vi "Finish.vi"(8 "error in (no error)":errorcluster, 11 "Compressor in":refnum<class "Compressor.lvclass">) -> (0 "error out":errorcluster, 3 "Compressor out":refnum<class "Compressor.lvclass">)   [LabVIEW 2013, in "Compressor.lvclass"]
uses:
  Compressor.lvclass
  System/System.lvclass
  Compressor.lvclass/Compressor.ctl
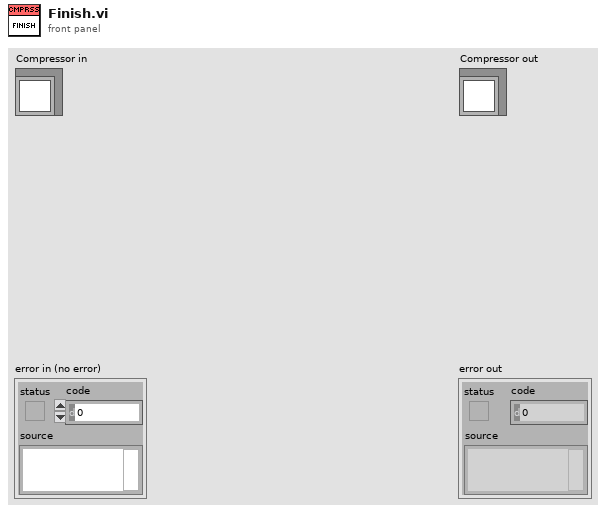
[diagram p1: front panel]
types:
  T1 = typedef "WPI_CompressorDevRef.ctl" = cluster{"DevStatus":errorcluster, "DigitalInputDevRef":T2, "RelayDevRef":T5}
  T2 = typedef "WPI_DigitalInputDevRef.ctl" = cluster{"DevStatus":errorcluster, "DIO Channel":T3, "Digital Module":T4}
  T3 = typedef "FPGA_DIOChannel.ctl" = enum8{"DIO 1", "DIO 2", "DIO 3", "DIO 4", "DIO 5", "DIO 6", "DIO 7", "DIO 8", "DIO 9", "DIO 10", "DIO 11", "DIO 12", "DIO 13", "DIO 14", "Invalid"}
  T4 = typedef "FPGA_TypedefDigitalModule.ctl" = enum16{"Digital Module 1", "Digital Module 2"}
  T5 = typedef "WPI_RelayDevRef.ctl" = cluster{"DevStatus":errorcluster, "Relay Channel":T6, "Digital Module":T4, "Relay Direction":T7}
  T6 = typedef "FPGA_DIORelayChannel.ctl" = enum8{"Relay 1", "Relay 2", "Relay 3", "Relay 4", "Relay 5", "Relay 6", "Relay 7", "Relay 8", "Invalid"}
  T7 = typedef "WPI_RelayDirection.ctl" = enum16{"Both directions", "Forward only", "Reverse only"}
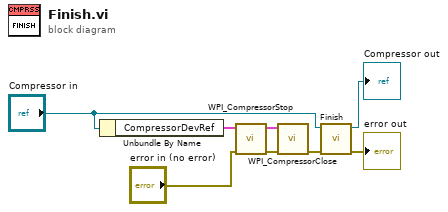
[diagram p0: block diagram]
diagram:
  n1 = Unbundle By Name("Compressor in") -> ("CompressorDevRef"=w3:T1)
  n2 = call <vilib>:"WPI_CompressorStop.vi"("error in (no error)"="error in (no error)", "CompressorDevRef"=w3) -> ("error out"=w6:errorcluster, "CompressorDevRef"=w5:T1)  [unwired: 8 in]
  n3 = call <vilib>:"WPI_CompressorClose.vi"("error in (no error)"=w6, "CompressorDevRef"=w5) -> ("error out"=w1:errorcluster)  [unwired: 9 in]
  n4 = call-parent "Finish.vi"("error in (no error)"=w1, "System in"="Compressor in") -> ("error out"=→"error out":errorcluster, "System out"=→"Compressor out":refnum<class "Compressor.lvclass">)  [unwired: 8 in]
